vi "Write Method Name.vi"(10 "Method Name":string, 11 "Abstract Message Scripter in":refnum<class "Abstract Message Scripter.lvclass">) -> (3 "Abstract Message Scripter out":refnum<class "Abstract Message Scripter.lvclass">)   [LabVIEW 2020, in "Message Maker.lvlib" / "Abstract Message Scripter.lvclass"]
uses:
  Abstract Message Scripter.lvclass
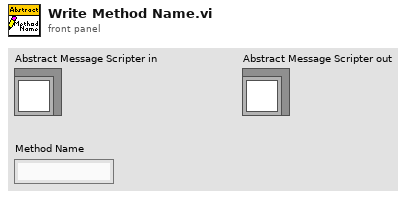
[diagram p1: front panel]
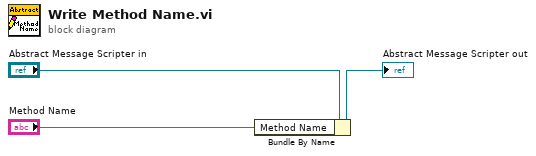
[diagram p0: block diagram]
diagram:
  n1 = Bundle By Name(cluster="Abstract Message Scripter in", "Method Name"="Method Name") -> (→"Abstract Message Scripter out":refnum<class "Abstract Message Scripter.lvclass">)
